vi "ProcessSerialData.vi"(8 "error in (no error)":errorcluster, 10 "Data in":string="SRNO=23234\nSOFT=40316\nXRT1=109\nSTAT=1089\nFREQ=170000\nSYNC=12345678\nEPOS=0\nDPOS=0\nINFO=2\nTIME=8427", 11 "Controller in":refnum<class "Controller.lvclass">) -> (0 "error out":errorcluster, 2 "Parsed Data":T1, 3 "Controller out":refnum<class "Controller.lvclass">)   [LabVIEW 2019, in "Controller.lvclass"]
uses:
  Controller.lvclass
  Serial parameters.ctl
  Controller.lvclass/Controller.ctl
panel:
  out "Stage types":string[][](array[string])
  out "Parameters":T2[](array[typedef])
  out "array":string[](array[string])
  # "Example data single axis"
  # "Example data multi axis"
  # "SRNO=23234\nSOFT=40316\nXRT1=109\nSTAT=1089\nFREQ=170000\nSYNC=12345678\nEPOS=0\nDPOS=0\nINFO=2\nTIME=8427"
  # "A:SRNO=0\nA:SOFT=40305\nA:XLS1=313\nA:STAT=17\nA:FREQ=170000\nA:SYNC=12345678\nA:EPOS=2\nA:DPOS=0\nA:PHAC=0\nA:TIME=55599\nB:SRNO=0\nB:SOFT=40305\nB:XLA1=312\nB:STAT=17\nB:FREQ=173000\nB:SYNC=12345678\nB:EPOS=1\nB:DPOS=0\nB:PROP=120\nB:TIME=29533\nC:SRNO=0\nC:SOFT=40305\nC:XRT1=109\nC:STAT=1\nC:FREQ=173000\nC:SYNC=12345678\nC:EPOS=0\nC:DPOS=0\nC:PROP=120\nC:TIME=30364\nD:SRNO=0\nD:SOFT=40305\nD:XLS3=1251\nD:STAT=401\nD:FREQ=87000\nD:SYNC=12345678\nD:EPOS=0\nD:DPOS=0\nD:PROP=120\nD:TIME=30387\nE:SRNO=0\nE:SOFT=40305\nE:XLA3=1250\nE:STAT=17\nE:FREQ=87000\nE:SYNC=12345678\nE:EPOS=0\nE:DPOS=0\nE:PROP=120\nE:TIME=30355"
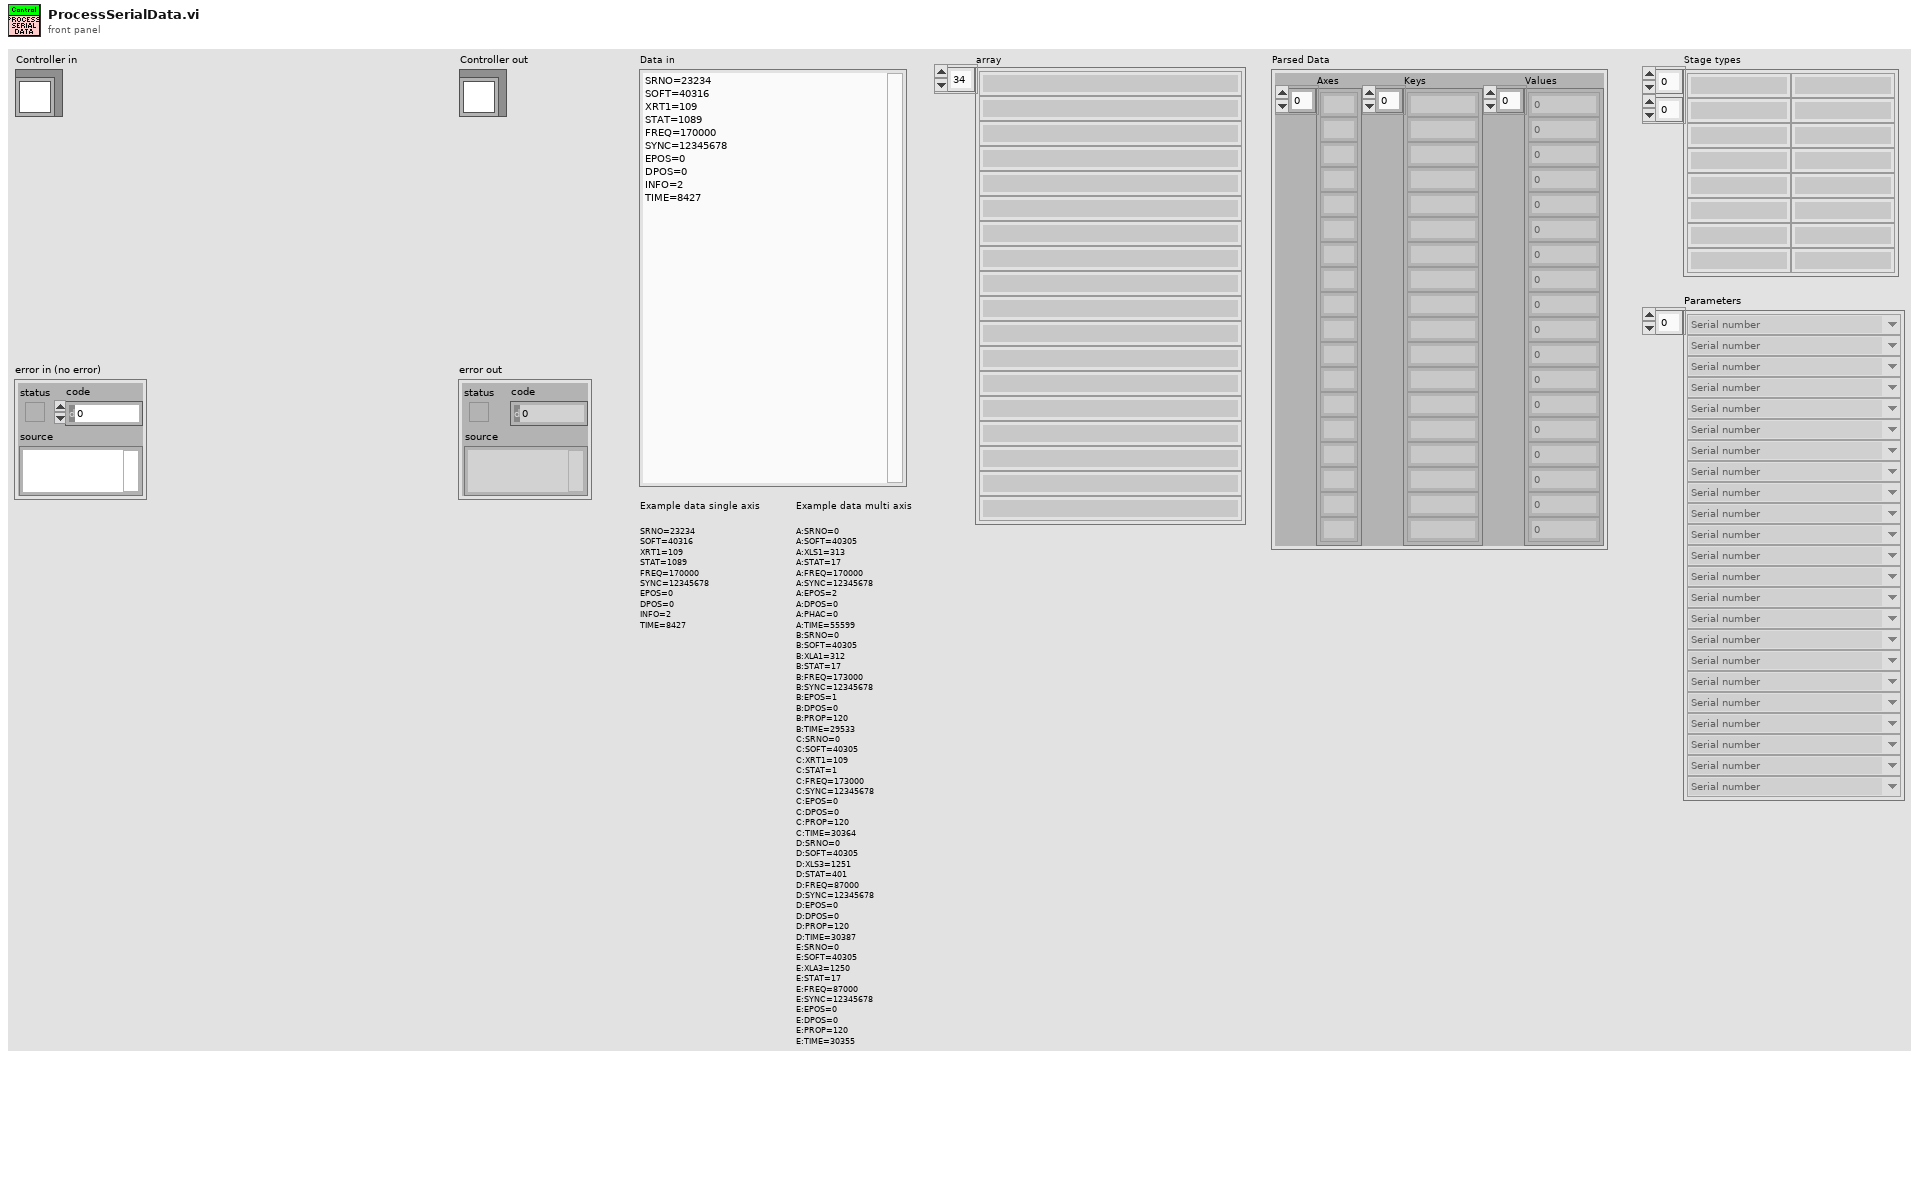
[diagram p1: front panel]
types:
  T1 = cluster{"Axes":string[], "Keys":string[], "Values":i32[]}
  T2 = typedef "Controller.lvclass/Serial parameters.ctl" = enum16{"Serial number", "Software number", "Type of stage", "Status", "Frequency", "Encoder position", "Desired position", "Info", "Phase correction", "Timestamp", "Proportional control factor", "Sync", "XRT1", "XRT3", "XRTA", "XLS1", "XLS3", "XLA1", "XLA3"}
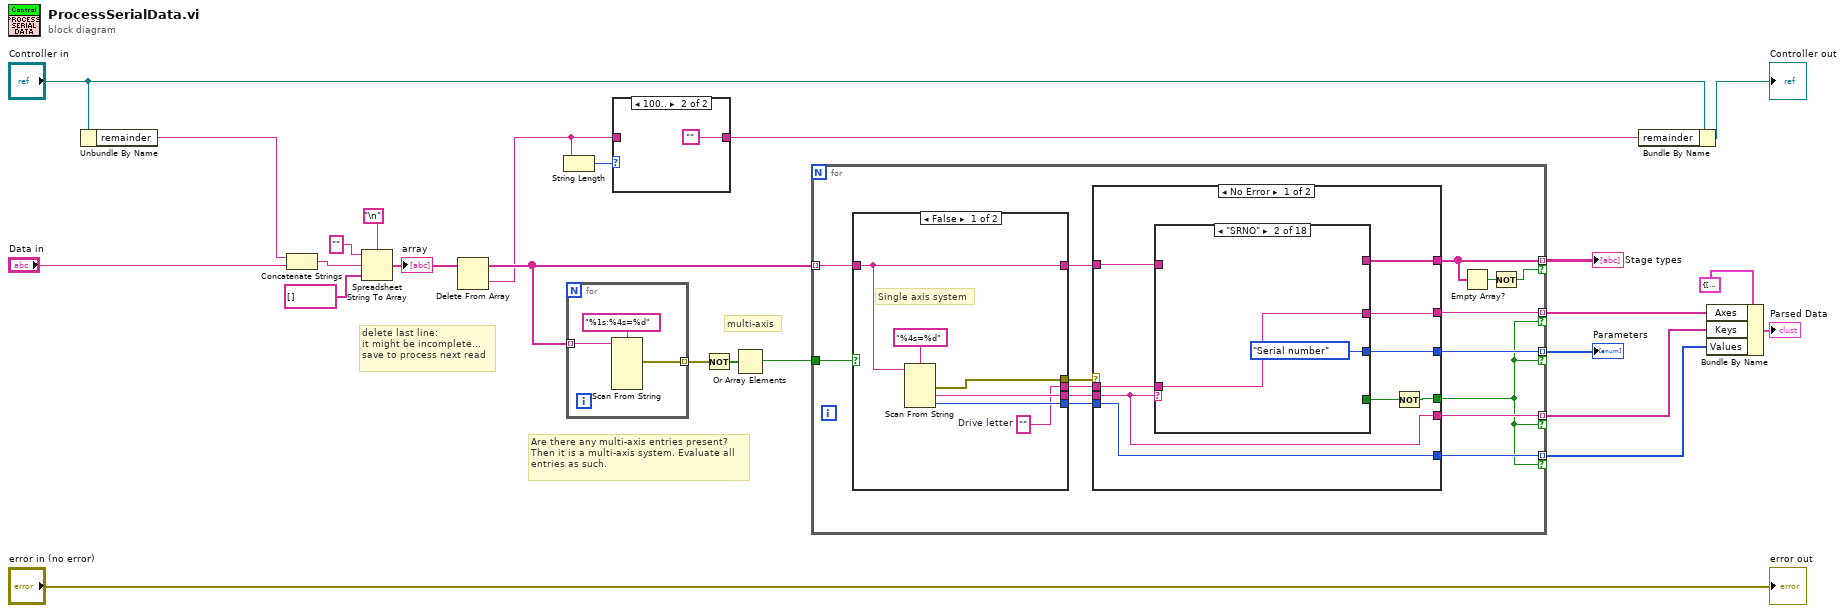
[diagram p0: block diagram]
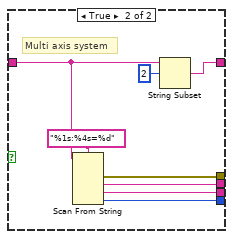
[diagram p3: hidden frame]
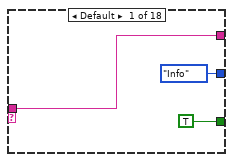
[diagram p4: hidden frame]
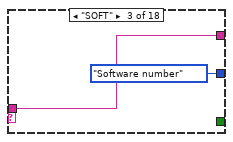
[diagram p5: hidden frame]
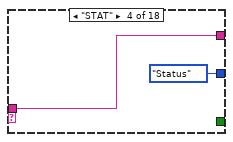
[diagram p6: hidden frame]
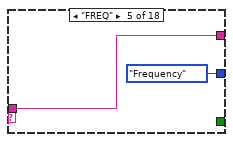
[diagram p7: hidden frame]
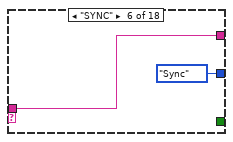
[diagram p8: hidden frame]
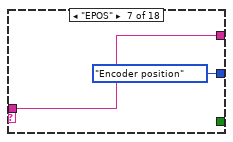
[diagram p9: hidden frame]
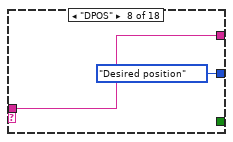
[diagram p10: hidden frame]
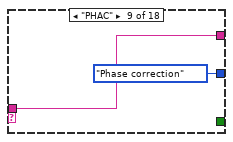
[diagram p11: hidden frame]
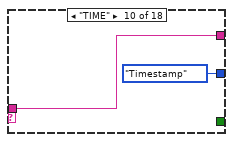
[diagram p12: hidden frame]
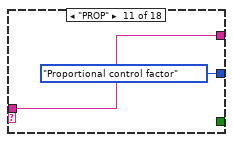
[diagram p13: hidden frame]
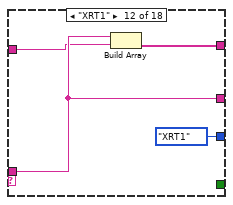
[diagram p14: hidden frame]
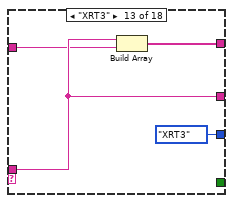
[diagram p15: hidden frame]
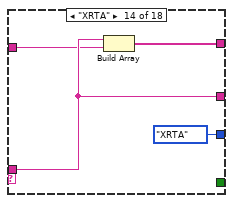
[diagram p16: hidden frame]
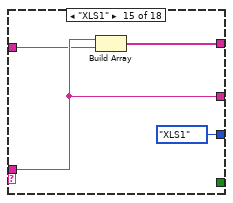
[diagram p17: hidden frame]
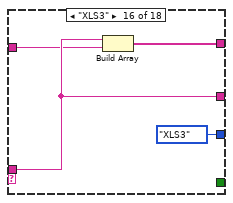
[diagram p18: hidden frame]
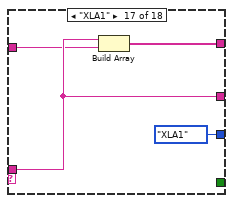
[diagram p19: hidden frame]
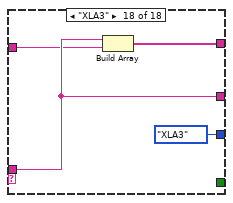
[diagram p20: hidden frame]
diagram:
  # "delete last line:\nit might be incomplete...\nsave to process next read"
  # "multi-axis"
  # "Are there any multi-axis entries present?\nThen it is a multi-axis system. Evaluate all\nentries as such."
  n1 = Unbundle By Name("Controller in") -> ("remainder"=w5:string)
  n2 = Concatenate Strings(w5, "Data in") -> (w11:string)
  n3 = Spreadsheet String To Array(delimiter (Tab)="\n", format string="", spreadsheet string=w11, array type (2D Dbl)=string[] []) -> (array=w10:string[])
  "array" <- w10
  n4 = Delete From Array(array=w10) -> (deleted portion=w3:string, array with subset deleted=w9:string[])  [unwired: 2 in]
  n5 = String Length(string=w3) -> (length=w4:i32)
  n6 = for {
    tunnel: w9 -> [w26] mode=indexing
    tunnel: [w25] -> w8 mode=indexing
    n7 = Scan From String(format string="%1s:%4s=%d", input string=w26) -> (error out=w25:errorcluster)  [unwired: 8 in, 2 out]
  }
  n8 = case shown="100.." w4 {
    tunnel: [w28 ""] -> w2
    tunnel: w3 -> [w28 _]
    frame Default {
    }
    frame 100.. {
    }
  }
  n9 = Not(x=w8) -> (.not. x?=w13:bool[])
  n10 = Or Array Elements(Boolean array=w13) -> (logical OR=w12:bool)
  n11 = for {
    tunnel: w9 -> [w42] mode=indexing
    tunnel: [w44] -> w24 mode=indexing if=w31
    tunnel: [w43] -> w19 mode=indexing if=w31
    tunnel: [w38] -> w21 mode=indexing if=w31
    tunnel: [w37] -> w23 mode=indexing if=w30
    tunnel: w12 -> [w35]
    tunnel: [w32] -> w20 mode=indexing if=w31
    n12 = case shown="False" w35 {
      tunnel: w42 -> [w45 w53]
      tunnel: [w49 w55] -> w41
      tunnel: [w48 w54] -> w40
      tunnel: [w47 w57] -> w39
      tunnel: [w46 w56] -> w34
      tunnel: [w45 w51] -> w33
      frame False {
        w46 = ""  # Drive letter
        # "Single axis system"
        n13 = Scan From String(format string="%4s=%d", input string=w45) -> (error out=w47:errorcluster, output 1=w49:string, output 2=w48:i32)  [unwired: 4 in, 2 out]
      }
      frame True {
        # "Multi axis system"
        n14 = Scan From String(format string="%1s:%4s=%d", input string=w53) -> (error out=w57:errorcluster, output 1=w56:string, output 2=w55:string, output 3=w54:i32)  [unwired: 5 in, 2 out]
        n15 = String Subset(string=w53, offset (0)=2) -> (substring=w51:string)  [unwired: 1 in]
      }
    }
    n16 = case shown="No Error" w39 {
      tunnel: [w61 _] -> w44
      tunnel: [w67 _] -> w43
      tunnel: [w60 _] -> w31
      tunnel: [w63 _] -> w37
      tunnel: w33 -> [w64 _]
      tunnel: w41 -> [w59 _]
      tunnel: w40 -> [w67 _]
      tunnel: [w62 _] -> w38
      tunnel: w34 -> [w65 _]
      tunnel: [w59 _] -> w32
      frame No Error {
        n17 = case shown="\"SRNO\"" w59 {
          tunnel: [Serial_parameters."Info" ("Enum") Serial_parameters."Serial number" ("Enum") Serial_parameters."Software number" ("Enum") Serial_parameters."Status" ("Enum") Serial_parameters."Frequency" ("Enum") Serial_parameters."Sync" ("Enum") Serial_parameters."Encoder position" ("Enum") Serial_parameters."Desired position" ("Enum") Serial_parameters."Phase correction" ("Enum") Serial_parameters."Timestamp" ("Enum") Serial_parameters."Proportional control factor" ("Enum") Serial_parameters."XRT1" ("Enum") Serial_parameters."XRT3" ("Enum") Serial_parameters."XRTA" ("Enum") Serial_parameters."XLS1" ("Enum") Serial_parameters."XLS3" ("Enum") Serial_parameters."XLA1" ("Enum") Serial_parameters."XLA3" ("Enum")] -> w61
          tunnel: [TRUE _ _ _ _ _ _ _ _ _ _ _ _ _ _ _ _ _] -> w66
          tunnel: w64 -> [_ _ _ _ _ _ _ _ _ _ _ w92 w96 w100 w104 w108 w112 w116]
          tunnel: [w68 w71 w73 w75 w77 w79 w81 w83 w85 w87 w89 w93 w97 w101 w105 w109 w113 w117] -> w62
          tunnel: w65 -> [w68 w71 w73 w75 w77 w79 w81 w83 w85 w87 w89 w93 w97 w101 w105 w109 w113 w117]
          tunnel: [_ _ _ _ _ _ _ _ _ _ _ w91 w95 w99 w103 w107 w111 w115] -> w63
          frame Default {
          }
          frame "SRNO" {
          }
          frame "SOFT" {
          }
          frame "STAT" {
          }
          frame "FREQ" {
          }
          frame "SYNC" {
          }
          frame "EPOS" {
          }
          frame "DPOS" {
          }
          frame "PHAC" {
          }
          frame "TIME" {
          }
          frame "PROP" {
          }
          frame "XRT1" {
            n18 = Build Array(w93, w92) -> (w91:string[])
          }
          frame "XRT3" {
            n19 = Build Array(w97, w96) -> (w95:string[])
          }
          frame "XRTA" {
            n20 = Build Array(w101, w100) -> (w99:string[])
          }
          frame "XLS1" {
            n21 = Build Array(w105, w104) -> (w103:string[])
          }
          frame "XLS3" {
            n22 = Build Array(w109, w108) -> (w107:string[])
          }
          frame "XLA1" {
            n23 = Build Array(w113, w112) -> (w111:string[])
          }
          frame "XLA3" {
            n24 = Build Array(w117, w116) -> (w115:string[])
          }
        }
        n25 = Not(x=w66) -> (.not. x?=w60:bool)
      }
      frame Error {
        # "unknown data. Discard."
      }
    }
    n26 = Empty Array?(array=w37) -> (empty?=w36:bool)
    n27 = Not(x=w36) -> (.not. x?=w30:bool)
  }
  "Parameters" <- w24
  "Stage types" <- w23
  n28 = Bundle By Name(cluster="Controller in", "remainder"=w2) -> (→"Controller out":refnum<class "Controller.lvclass">)
  n29 = Bundle By Name(cluster=T1 {"Axes"=[], "Keys"=[], "Values"=[]} ("Parsed Data"), "Axes"=w21, "Keys"=w20, "Values"=w19) -> (→"Parsed Data":T1)
  "error out" <- "error in (no error)"
